vi "Main.vi"() -> ()   [LabVIEW 2016]
doc: "The roboRIO Project template acquires acceleration data from the onboard accelerometer and displays the changes of acceleration values in a waveform chart."
uses:
  <vilib>/myRIO/Instrument Drivers/Onboard IO/DIO/typedefs/DIO Reference.ctl
  <vilib>/myRIO/Common/Instrument Driver Framework/Utilities/typedefs/myRIO Generic Hardware Reference.ctl
  <vilib>/myRIO/Common/Instrument Driver Framework/Utilities/typedefs/Hardware Version Enum.ctl
  <vilib>/myRIO/Common/Instrument Driver Framework/Utilities/typedefs/myRIO v1.0 Reference.ctl
  <vilib>/myRIO/Common/Instrument Driver Framework/Utilities/typedefs/Generic FPGA Reference.ctl
  <vilib>/myRIO/Common/Instrument Driver Framework/myRIO v1.0/DIO/typedefs/DIO Channels List.ctl
  <vilib>/myRIO/Common/Instrument Driver Framework/myRIO v1.0/DIO/typedefs/DIO Channels Enum.ctl
  <vilib>/userdefined/High Color/nirio_resource_hc.ctl
  <vilib>/myRIO/Common/Instrument Driver Framework/Utilities/vis/Is FPGA Ref Available.vi
  <vilib>/myRIO/Common/Instrument Driver Framework/roboRIO v1.0/DIO/vis/roboRIO v1.0 Open DIO.vi
  <vilib>/myRIO/Instrument Drivers/Onboard IO/DIO/vis/Write.vi
  <vilib>/myRIO/Instrument Drivers/Onboard IO/DIO/vis/Read.vi
  <vilib>/myRIO/Common/Instrument Driver Framework/Utilities/vis/Validate Channels.vi
  <vilib>/myRIO/Common/Instrument Driver Framework/roboRIO v1.0/DIO/vis/roboRIO v1.0 Reserve DIO.vi
  <vilib>/myRIO/Common/Instrument Driver Framework/roboRIO v1.0/DIO/vis/roboRIO v1.0 Build MUX Configuration DIO.vi
  <vilib>/myRIO/Common/Instrument Driver Framework/roboRIO v1.0/Resource Manager/vis/roboRIO v1.0 Reserve Channel List.vi
  <vilib>/myRIO/Common/Instrument Driver Framework/roboRIO v1.0/Resource Manager/vis/roboRIO v1.0 Create Configuration List.vi
  <vilib>/myRIO/Common/Instrument Driver Framework/roboRIO v1.0/Resource Manager/vis/roboRIO v1.0 Reserve Channel.vi
  <vilib>/myRIO/Common/Instrument Driver Framework/roboRIO v1.0/Resource Manager/vis/roboRIO v1.0 Unreserve Channel.vi
  <vilib>/myRIO/Common/Instrument Driver Framework/roboRIO v1.0/Resource Manager/vis/roboRIO v1.0 Build Mutex Name.vi
  <vilib>/FPGAPlugInAG/roboRIO/niLvFpga_Open_roboRIO.vi
  <vilib>/rvi/interface/common/dynamic/niFpgaDynamicAddResources.vi
  <vilib>/FPGAPlugInAG/Dynamic/niLvFpga_Reset_Dynamic.vi
  <vilib>/myRIO/Common/Instrument Driver Framework/Utilities/vis/FPGA Ref Manager.vi
  builds/UnicornMain/UnicornRIO1/ROS for LabVIEW/home/lvuser/natinst/bin/vi.lib/Utility/error.llb/Error Cluster From Error Code.vi
  <vilib>/myRIO/Common/Instrument Driver Framework/Utilities/vis/Ref Counter.vi
  <vilib>/FPGAPlugInAG/Dynamic/niLvFpga_Run_Dynamic.vi
  UnicornMain/GlobalVI.vi
  builds/ROS_Test1/UnicornRIO1/ROS for LabVIEW/home/lvuser/natinst/bin/user.lib/ROS for LabVIEW Software/ROS/Code/_ROSDefinition.vi
  UnicornMain/Global 2.vi
  <vilib>/Utility/VariantDataType/GetNumericInfo.vi
  <vilib>/myRIO/Common/Instrument Driver Framework/roboRIO v1.0/roboRIO v1.0 Open.vi
  <vilib>/myRIO/Common/Instrument Driver Framework/Utilities/vis/IO Manager.vi
  <vilib>/myRIO/Common/Instrument Driver Framework/Utilities/vis/Configuration Manager.vi
  <vilib>/myRIO/Common/Instrument Driver Framework/roboRIO v1.0/Resource Manager/vis/roboRIO v1.0 Configure IO.vi
  <vilib>/myRIO/Common/Instrument Driver Framework/myRIO v1.0/myRIO v1.0 Close.vi
  <vilib>/myRIO/Common/Instrument Driver Framework/roboRIO v1.0/DIO/vis/roboRIO v1.0 Read DIO.vi
  <vilib>/myRIO/Common/Instrument Driver Framework/roboRIO v1.0/DIO/vis/roboRIO v1.0 Write DIO.vi
  <vilib>/FPGAPlugInAG/Dynamic/niLvFpga_Close_Dynamic.vi
  <vilib>/rvi/interface/nirviOpenFPGA/nirviOpenFPGA.xnode
  UnicornMain/FPGA/FPGA Bitfiles/UnicornMain_FPGATarget_MainFPGAcode_pijQzTnE6Wg.lvbitx
  <vilib>/rvi/interface/nirviMethod/nirviMethod.xnode
  <vilib>/myRIO/Express VI/Onboard Devices/Button/Button Express VI.xnode
  <vilib>/myRIO/Instrument Drivers/Onboard IO/DIO/vis/myRIO DIO Open.xnode
  <vilib>/myRIO/Express VI/Onboard Devices/LED/LED Express VI.xnode
  <vilib>/rvi/interface/nirviCloseFPGA/nirviCloseFPGA.xnode
  <vilib>/myRIO/Instrument Drivers/Utilities/Utilities.lvlib
  <vilib>/FPGAPlugInAG/Dynamic/niLvFpga_StartFifo_Dynamic.vi
  <vilib>/rvi/errors/niLvFpgaMergeErrorWithErrorCode.vi
  <vilib>/myRIO/Instrument Drivers/Onboard IO/DIO/DIO.lvlib
panel:
  out "runLiftStatemachine 2":bool
  out "x 2":dbl
  out "y 2":dbl
  out "z 2":dbl
  out "runLidarBack 2":bool
  out "Emergency STOP 2":bool
  out "Sytem Online 2":bool
  out "currentDirection 2":i32
  out "timeout 2":u32
  out "StartTime 2":u32
  out "FPGA REF Error out 2":errorcluster
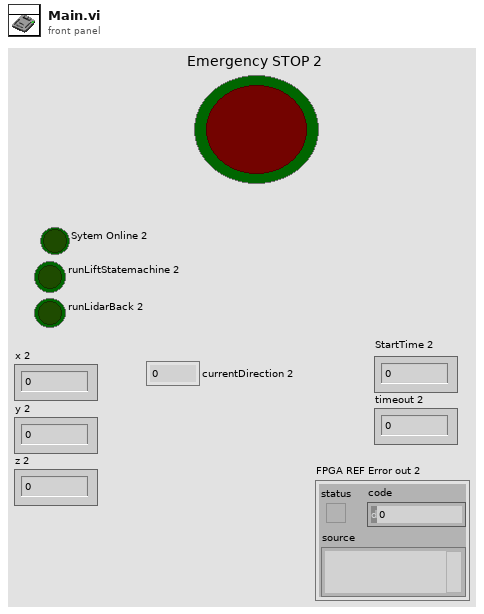
[diagram p1: front panel]
types:
  T1 = typedef "DIO.lvlib/DIO Reference.ctl" = cluster{"myRIO Reference":T2, "DIO Channels List":T6}
  T2 = typedef "myRIO Generic Hardware Reference.ctl" = cluster{"myRIO Model":T3, "myRIO Hardware Reference":T4}
  T3 = typedef "Hardware Version Enum.ctl" = enum16{"Unknown", "myRIO-1900", "myRIO-1950", "roboRIO", "NI ELVIS RIO CM"}
  T4 = typedef "myRIO v1.0 Reference.ctl" = cluster{"Generic FPGA Reference":T5, "Allow multiple opens":bool}
  T5 = typedef "Generic FPGA Reference.ctl" = refnum<k20>
  T6 = typedef "DIO Channels List.ctl" = T7[]
  T7 = typedef "DIO Channels Enum.ctl" = enum16{"Not Connected", "C/DIO0", "C/DIO1", "C/DIO2", "C/DIO3", "C/DIO4", "C/DIO5", "C/DIO6", "C/DIO7", "A/DIO0", "A/DIO1", "A/DIO2", "A/DIO3", "A/DIO4", "A/DIO5", "A/DIO6", "A/DIO7", "A/DIO8", "A/DIO9", "A/DIO10", "A/DIO11", "A/DIO12", "A/DIO13", "A/DIO14", "A/DIO15", "B/DIO0", "B/DIO1", "B/DIO2", "B/DIO3", "B/DIO4", "B/DIO5", "B/DIO6", "B/DIO7", "B/DIO8", "B/DIO9", "B/DIO10", "B/DIO11", "B/DIO12", "B/DIO13", "B/DIO14", "B/DIO15", "LED0", "LED1", "LED2", "LED3", "Button0", "DIO/DIO0", "DIO/DIO1", "DIO/DIO2", "DIO/DIO3", "DIO/DIO4", "DIO/DIO5", "DIO/DIO6", "DIO/DIO7", "DIO/DIO8", "DIO/DIO9", "SPI/CS0", "SPI/CS1", "SPI/CS2", "SPI/CS3", "LED RADIO (Green)", "LED RADIO (Red)", "LED COMM (Green)", "LED COMM (Red)", "LED MODE (Green)", "LED MODE (Red)"}
  T8 = typedef "nirio_resource_hc.ctl" = tag
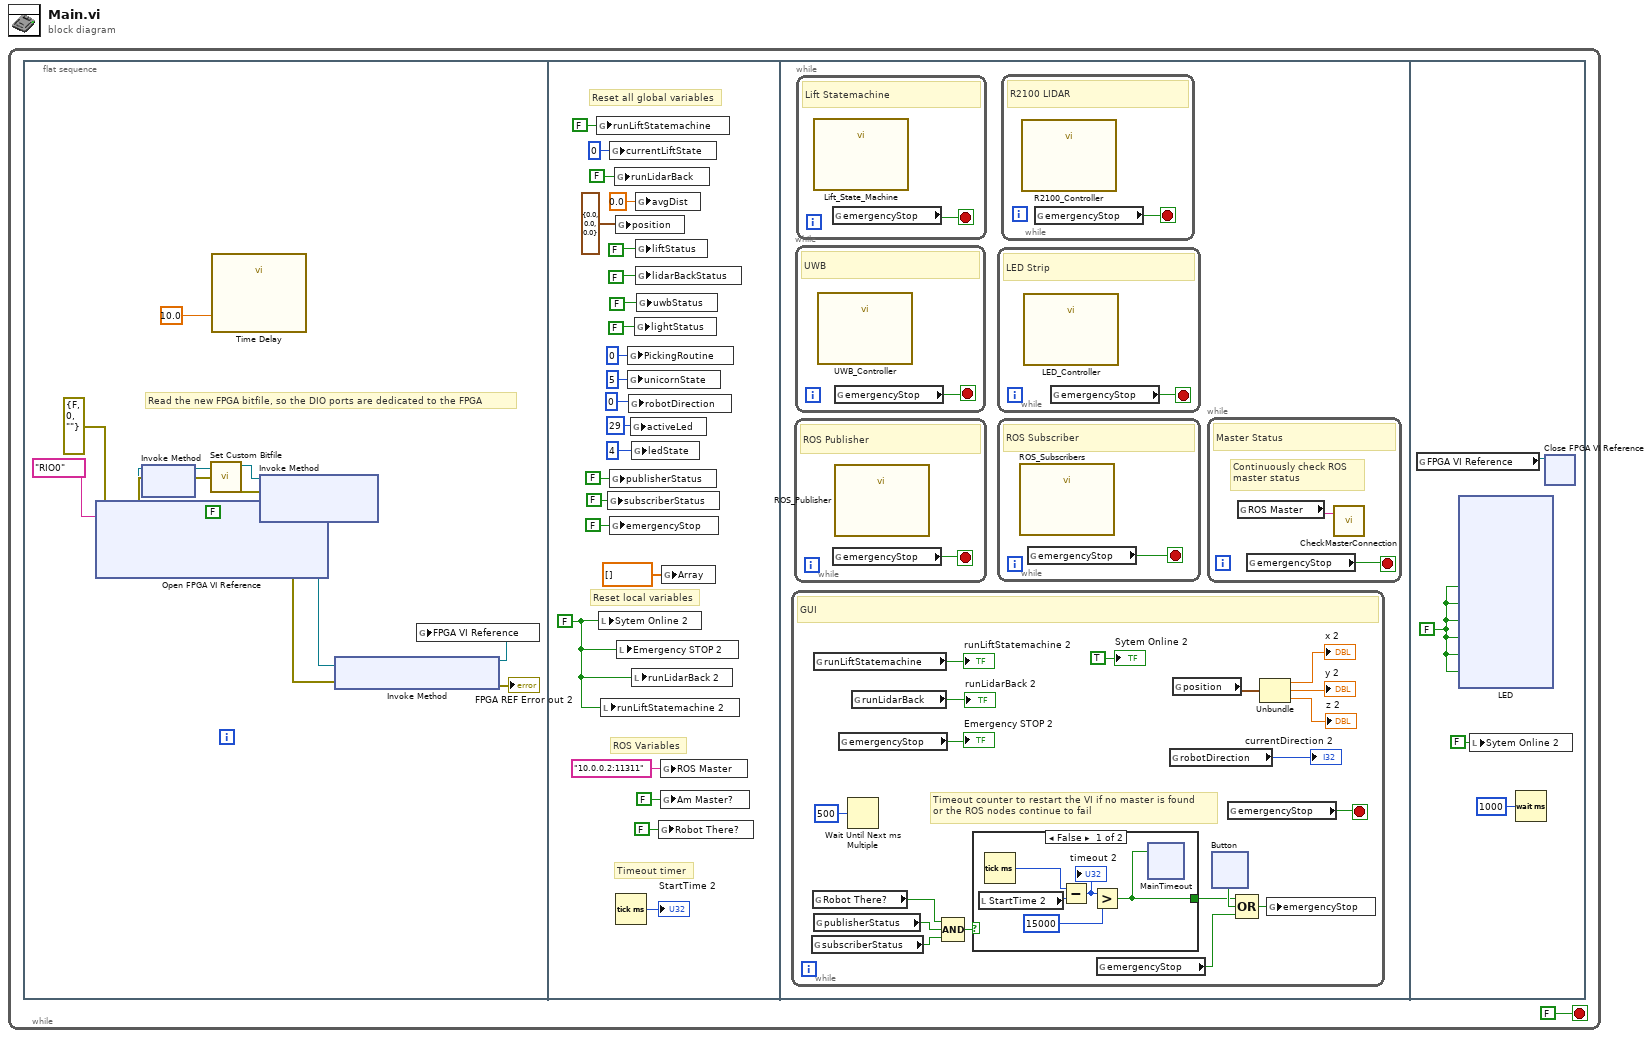
[diagram p0: block diagram]
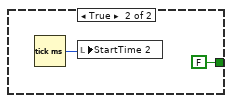
[diagram p2: hidden frame]
diagram:
  n1 = while {
    stop <- FALSE stop-if-true
    n2 = flat-sequence {
      frame #0 {
        # "Read the new FPGA bitfile, so the DIO ports are dedicated to the FPGA"
        n3 = xnode "Open FPGA VI Reference"("error in"=errorcluster {"status"=FALSE, "code"=0, "source"=""}, "resource name"=tag "RIO0") -> ("FPGA VI Reference Out"=w8:refnum<k20>, "error out"=w9:errorcluster)
        n4 = xnode "Invoke Method"("FPGA VI Reference In"=w8, "error in"=w9) -> ("FPGA VI Reference Out"=w12:refnum<k20>, "error out"=w11:errorcluster)
        n5 = call <vilib>:"Set Custom Bitfile.vi"("error in (no error)"=w11, "Custom FPGA Reference In"=w12) -> ("error out"=w13:errorcluster, "Custom FPGA Reference Out"=w14:refnum<k20>)  [unwired: 8 in]
        n6 = call "Time Delay"("Delay Time (s)"=10.0) -> ()  [unwired: 10 in, 1 out]
        n7 = xnode "Invoke Method"("FPGA VI Reference In"=w14, "error in"=w13, "Wait Until Done (F)"=FALSE) -> ("FPGA VI Reference Out"=w6:refnum<k20>, "error out"=w5:errorcluster)
        n8 = xnode "Invoke Method"("FPGA VI Reference In"=w6, "error in"=w5) -> ("FPGA VI Reference Out"=w4:refnum<k20>, "error out"=→"FPGA REF Error out 2":errorcluster)
        n9 = global write "GlobalVI.vi" "FPGA VI Reference"(w4) -> ()
      }
      frame #1 {
        w30 = FALSE ("Sytem Online")
        # "Timeout timer"
        # "ROS Variables"
        # "Reset local variables"
        # "Reset all global variables"
        n10 = global write "GlobalVI.vi" "runLiftStatemachine"(FALSE ("runLiftStatemachine")) -> ()
        n11 = local write "Sytem Online 2"(w30) -> ()
        n12 = local write "runLiftStatemachine 2"(w30) -> ()
        n13 = global write "GlobalVI.vi" "subscriberStatus"(FALSE ("subscriberStatus")) -> ()
        n14 = global write "GlobalVI.vi" "currentLiftState"(0 ("currentLiftState")) -> ()
        n15 = global write "GlobalVI.vi" "publisherStatus"(FALSE ("publisherStatus")) -> ()
        n16 = global write "GlobalVI.vi" "emergencyStop"(FALSE ("emergencyStop")) -> ()
        n17 = global write "GlobalVI.vi" "runLidarBack"(FALSE ("runLidarBack")) -> ()
        n18 = global write "GlobalVI.vi" "position"(cluster{"x":dbl, "y":dbl, "z":dbl} {"x"=0.0, "y"=0.0, "z"=0.0} ("position")) -> ()
        n19 = Tick Count (ms)() -> (millisecond timer value=→"StartTime 2":u32)
        n20 = local write "Emergency STOP 2"(w30) -> ()
        n21 = global write "GlobalVI.vi" "PickingRoutine"(0 ("PickingRoutine")) -> ()
        n22 = global write "GlobalVI.vi" "unicornState"(5 ("unicornState")) -> ()
        n23 = global write "GlobalVI.vi" "robotDirection"(0 ("robotDirection")) -> ()
        n24 = global write "GlobalVI.vi" "activeLed"(29 ("activeLed")) -> ()
        n25 = global write "GlobalVI.vi" "ledState"(4 ("ledState")) -> ()
        n26 = local write "runLidarBack 2"(w30) -> ()
        n27 = global write "GlobalVI.vi" "lightStatus"(FALSE ("lightStatus")) -> ()
        n28 = global write "GlobalVI.vi" "avgDist"(sgl 0.0 ("avgDist")) -> ()
        n29 = global write "GlobalVI.vi" "liftStatus"(FALSE ("liftStatus")) -> ()
        n30 = global write "GlobalVI.vi" "lidarBackStatus"(FALSE ("lidarBackStatus")) -> ()
        n31 = global write "GlobalVI.vi" "uwbStatus"(FALSE ("uwbStatus")) -> ()
        n32 = global write "_ROSDefinition.vi" "Robot There?"(FALSE ("Robot There?")) -> ()
        n33 = global write "_ROSDefinition.vi" "ROS Master"("10.0.0.2:11311" ("ROS Master")) -> ()
        n34 = global write "_ROSDefinition.vi" "Am Master?"(FALSE ("Am Master?")) -> ()
        n35 = global write "Global 2.vi" "Array"(dbl[] [] ("Array")) -> ()
      }
      frame #2 {
        n36 = while {
          stop <- w59 stop-if-true
          # "Timeout counter to restart the VI if no master is found\nor the ROS nodes continue to fail"
          # "GUI"
          n37 = global read "GlobalVI.vi" "subscriberStatus"() -> (w49:bool)
          n38 = global read "_ROSDefinition.vi" "Robot There?"() -> (w51:bool)
          n39 = global read "GlobalVI.vi" "runLiftStatemachine"() -> (→"runLiftStatemachine 2":bool)
          n40 = global read "GlobalVI.vi" "publisherStatus"() -> (w50:bool)
          n41 = global read "GlobalVI.vi" "emergencyStop"() -> (→"Emergency STOP 2":bool)
          n42 = Wait Until Next ms Multiple(millisecond multiple=u32 500) -> ()  [unwired: 1 out]
          n43 = global read "GlobalVI.vi" "runLidarBack"() -> (→"runLidarBack 2":bool)
          n44 = Compound Arithmetic op=AND(w51, w50, w49) -> (w48:bool)
          n45 = case shown="False" w48 {
            tunnel: [w65 FALSE] -> w52
            frame False {
              n46 = local read "StartTime 2"() -> (w69:u32)
              n47 = Tick Count (ms)() -> (millisecond timer value=w68:u32)
              n48 = Subtract(x=w68, y=w69) -> (x-y=w67:u32)
              "timeout 2" <- w67
              n49 = Greater?(x=w67, y=u32 15000) -> (0:w65:bool)
              n50 = xnode ("MainTimeout")("RADIO (Red)"=w65) -> ()  [unwired: 1 in, 1 out]
            }
            frame True {
              n51 = Tick Count (ms)() -> (millisecond timer value=w105:u32)
              n52 = local write "StartTime 2"(w105) -> ()
            }
          }
          n53 = global read "GlobalVI.vi" "emergencyStop"() -> (w46:bool)
          n54 = global read "GlobalVI.vi" "robotDirection"() -> (→"currentDirection 2":i32)
          n55 = global read "GlobalVI.vi" "position"() -> (w63:cluster{"x":dbl, "y":dbl, "z":dbl})
          n56 = xnode "Button"() -> ("Value"=w53:bool)  [unwired: 1 in, 1 out]
          n57 = global read "GlobalVI.vi" "emergencyStop"() -> (w59:bool)
          n58 = Compound Arithmetic op=OR(w52, w53, w46) -> (w47:bool)
          n59 = Unbundle(w63) -> ("x"=→"x 2":dbl, "y"=→"y 2":dbl, "z"=→"z 2":dbl)
          n60 = global write "GlobalVI.vi" "emergencyStop"(w47) -> ()
          "Sytem Online 2" <- TRUE ("Sytem Online")
        }
        n61 = while {
          stop <- w43 stop-if-true
          # "ROS Publisher"
          n62 = global read "GlobalVI.vi" "emergencyStop"() -> (w43:bool)
          n63 = call "ROS_Publisher.vi"() -> ()  [unwired: 12 in]
        }
        n64 = while {
          stop <- w39 stop-if-true
          # "UWB"
          n65 = call "UWB_Controller.vi"() -> ()  [unwired: 12 in]
          n66 = global read "GlobalVI.vi" "emergencyStop"() -> (w39:bool)
        }
        n67 = while {
          stop <- w142 stop-if-true
          # "Lift Statemachine"
          n68 = call "Lift_State_Machine.vi"() -> ()  [unwired: 12 in]
          n69 = global read "GlobalVI.vi" "emergencyStop"() -> (w142:bool)
        }
        n70 = while {
          stop <- w42 stop-if-true
          # "LED Strip"
          n71 = call "LED_Controller.vi"() -> ()  [unwired: 12 in]
          n72 = global read "GlobalVI.vi" "emergencyStop"() -> (w42:bool)
        }
        n73 = while {
          stop <- w44 stop-if-true
          # "ROS Subscriber"
          n74 = call "ROS_Subscribers.vi"() -> ()  [unwired: 12 in]
          n75 = global read "GlobalVI.vi" "emergencyStop"() -> (w44:bool)
        }
        n76 = while {
          stop <- w45 stop-if-true
          # "R2100 LIDAR"
          n77 = call "R2100_Controller.vi"() -> ()  [unwired: 11 in]
          n78 = global read "GlobalVI.vi" "emergencyStop"() -> (w45:bool)
        }
        n79 = while {
          stop <- w40 stop-if-true
          # "Continuously check ROS\nmaster status"
          # "Master Status"
          n80 = global read "_ROSDefinition.vi" "ROS Master"() -> (w41:string)
          n81 = global read "GlobalVI.vi" "emergencyStop"() -> (w40:bool)
          n82 = call "CheckMasterConnection.vi"("Master IP"=w41) -> ()  [unwired: 1 in, 2 out]
        }
      }
      frame #3 {
        w146 = FALSE
        n83 = global read "GlobalVI.vi" "FPGA VI Reference"() -> (w144:refnum<k20>)
        n84 = xnode "LED"("RADIO (Green)"=w146, "RADIO (Red)"=w146, "COMM (Green)"=w146, "COMM (Red)"=w146, "MODE (Green)"=w146, "MODE (Red)"=w146) -> ()  [unwired: 1 in, 1 out]
        n85 = local write "Sytem Online 2"(FALSE ("Sytem Online")) -> ()
        n86 = Wait (ms)(milliseconds to wait=u32 1000) -> ()  [unwired: 1 out]
        n87 = xnode "Close FPGA VI Reference"("FPGA VI Reference In"=w144) -> ()  [unwired: 1 in, 1 out]
      }
    }
  }
